vi "PathPlanner_PathFinder_GNotFound.vi"   [LabVIEW 2019]
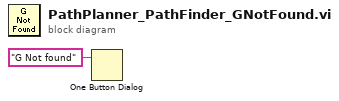
[diagram p0: block diagram]
diagram:
  n1 = One Button Dialog(message="G Not found") -> ()  [unwired: 1 in, 1 out]
